vi "Setup.vi"(11 "Base Queue jettl in":refnum<class "Base Queue jettl.lvclass">) -> (3 "Base Queue jettl out":refnum<class "Base Queue jettl.lvclass">)   [LabVIEW 2021, in "jettl.lvlib" / "Base Queue jettl.lvlib" / "Base Queue jettl.lvclass"]
uses:
  Base Queue jettl.lvclass
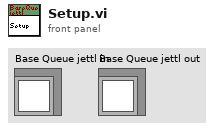
[diagram p1: front panel]
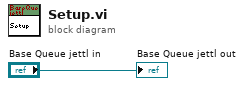
[diagram p0: block diagram]
diagram:
  "Base Queue jettl out" <- "Base Queue jettl in"
